vi "calculateChecksum.vi"(0 "Initial Command":string, 11 "error in (no error)":errorcluster) -> (2 "ADDR 1":string, 3 "ADDR 2":string, 4 "COMM 1":string, 6 "COMM 2":string, 8 "DATA 1":string, 10 "DATA 2":string, 13 "CHECKSUM":string, 14 "Start bit + Command + Check Sum + 2 Stop bits":string, 15 "error out":errorcluster)   [LabVIEW 2018]
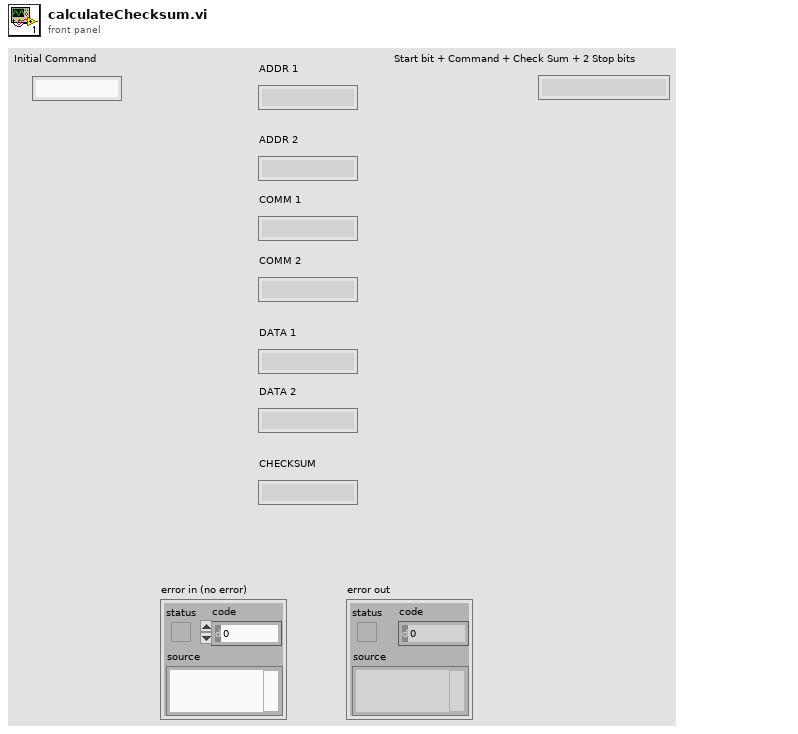
[diagram p1: front panel]
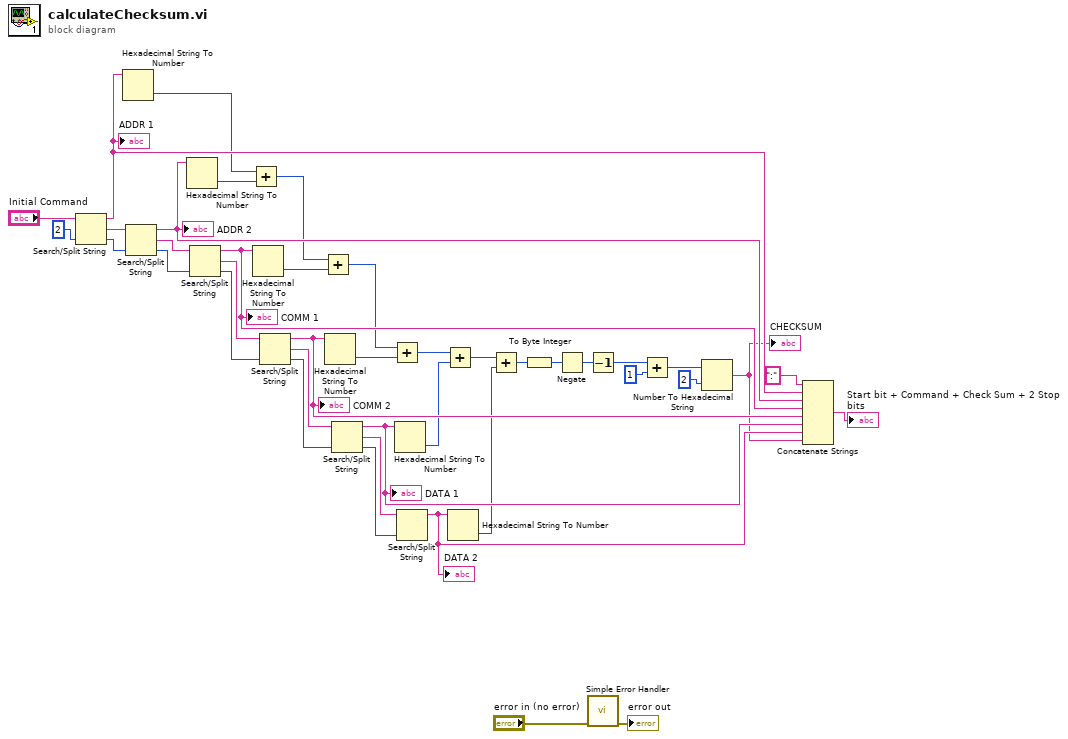
[diagram p0: block diagram]
diagram:
  n1 = Search/Split String(string="Initial Command", offset (0)=2) -> (substring before match=w33:string, match + rest of string=w24:string, offset of match=w23:i32)  [unwired: 1 in]
  "ADDR 1" <- w33
  n2 = Hexadecimal String To Number(string=w33) -> (number=w1:u32)  [unwired: 2 in, 1 out]
  n3 = Search/Split String(string=w24, offset (0)=w23) -> (substring before match=w34:string, match + rest of string=w26:string, offset of match=w25:i32)  [unwired: 1 in]
  "ADDR 2" <- w34
  n4 = Hexadecimal String To Number(string=w34) -> (number=w2:u32)  [unwired: 2 in, 1 out]
  n5 = Search/Split String(string=w26, offset (0)=w25) -> (substring before match=w35:string, match + rest of string=w28:string, offset of match=w27:i32)  [unwired: 1 in]
  "COMM 1" <- w35
  n6 = Add(x=w1, y=w2) -> (x+y=w4:u32)
  n7 = Hexadecimal String To Number(string=w35) -> (number=w3:u32)  [unwired: 2 in, 1 out]
  n8 = Search/Split String(string=w28, offset (0)=w27) -> (substring before match=w36:string, match + rest of string=w30:string, offset of match=w29:i32)  [unwired: 1 in]
  "COMM 2" <- w36
  n9 = Add(x=w4, y=w3) -> (x+y=w5:u32)
  n10 = Hexadecimal String To Number(string=w36) -> (number=w6:u32)  [unwired: 2 in, 1 out]
  n11 = Search/Split String(string=w30, offset (0)=w29) -> (substring before match=w37:string, match + rest of string=w32:string, offset of match=w31:i32)  [unwired: 1 in]
  "DATA 1" <- w37
  n12 = Add(x=w5, y=w6) -> (x+y=w7:u32)
  n13 = Hexadecimal String To Number(string=w37) -> (number=w8:u32)  [unwired: 2 in, 1 out]
  n14 = Search/Split String(string=w32, offset (0)=w31) -> (substring before match=w38:string)  [unwired: 1 in, 2 out]
  "DATA 2" <- w38
  n15 = Add(x=w7, y=w8) -> (x+y=w9:u32)
  n16 = Hexadecimal String To Number(string=w38) -> (number=w10:u32)  [unwired: 2 in, 1 out]
  n17 = Add(x=w9, y=w10) -> (x+y=w11:u32)
  n18 = To Byte Integer(number=w11) -> (8bit integer=w13:i8)
  n19 = Negate(x=w13) -> (-x=w12:i8)
  n20 = Decrement(x=w12) -> (x-1=w14:i8)
  n21 = call <vilib>:"Simple Error Handler.vi"("error in (no error)"="error in (no error)") -> ("error out"=→"error out":errorcluster)  [unwired: 4 in, 4 out]
  n22 = Add(x=w14, y=i8 1) -> (x+y=w16:i8)
  n23 = Number To Hexadecimal String(1:i16 2 ("width (-)"), 2:w16) -> (0:w19:string)
  "CHECKSUM" <- w19
  n24 = Concatenate Strings(":" ("START 0"), w33, w34, w35, w36, w37, w38, w19) -> (→"Start bit + Command + Check Sum + 2 Stop bits":string)
